vi "Configure Server.vi"(8 "error in (no error)":errorcluster, 9 "server configuration":cluster{"enabled":bool}, 10 "server index":u16, 11 "PLBB in":refnum<class "PL BlackBox Modbus Client.lvclass">) -> (0 "error out":errorcluster, 3 "PLBB out":refnum<class "PL BlackBox Modbus Client.lvclass">)   [LabVIEW 2015, in "PL BlackBox Modbus Client.lvclass"]
doc: "Configures the server."
uses:
  PL BlackBox Modbus Client.lvclass
  <vilib>/plasmapper/PL Modbus Client/PL Modbus Client.lvclass
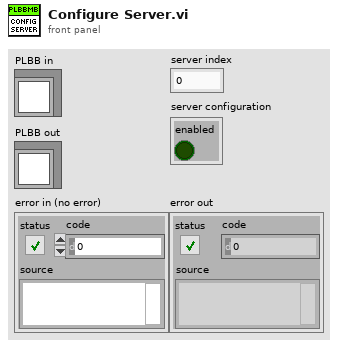
[diagram p1: front panel]
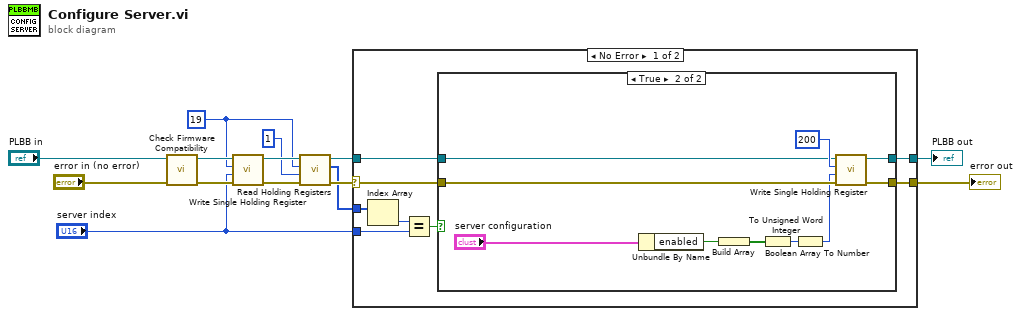
[diagram p0: block diagram]
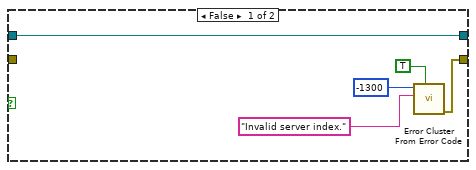
[diagram p2: hidden frame]
diagram:
  w6 = u16 19 ("address")
  n1 = call-dynamic "Check Firmware Compatibility.vi"("error in (no error)"="error in (no error)", "PLBB in"="PLBB in") -> ("error out"=w9:errorcluster, "PLBB out"=w10:refnum<class "PL BlackBox Modbus Client.lvclass">)  [unwired: 8 in]
  n2 = call <vilib>:"Write Single Holding Register.vi"("error in (no error)"=w9, "value"="server index", "address"=w6, "MODBUS in"=w10) -> ("error out"=w5:errorcluster, "MODBUS out"=w8:refnum<class "PL BlackBox Modbus Client.lvclass">)  [unwired: 6 in]
  n3 = call <vilib>:"Read Holding Registers.vi"("error in (no error)"=w5, "number of holding registers"=u16 1 ("address"), "address"=w6, "MODBUS in"=w8) -> ("error out"=w4:errorcluster, "values"=w2:u16[], "MODBUS out"=w3:refnum<class "PL BlackBox Modbus Client.lvclass">)  [unwired: 5 in]
  n4 = case shown="No Error" w4 {
    selector: w4 -> [w16 w38]
    tunnel: [w22 w38] -> w14
    tunnel: [w21 w39] -> w13
    tunnel: w3 -> [w17 w39]
    tunnel: w2 -> [w20 _]
    tunnel: "server index" -> [w15 _]
    frame No Error {
      n5 = Index Array(array=w20) -> (element=w19:u16)  [unwired: 1 in]
      n6 = Equal?(x=w19, y=w15) -> (x = y?=w18:bool)
      n7 = case shown="True" w18 {
        tunnel: [w23 w36] -> w22
        tunnel: [w27 w37] -> w21
        tunnel: w17 -> [w27 w30]
        tunnel: w16 -> [_ w29]
        frame False {
          n8 = call <vilib>:"Error Cluster From Error Code.vi"("show call chain? (False)"=TRUE, "error message (\"\")"="Invalid server index." ("error message (\"\")"), "error code (0)"=-1300) -> ("error out"=w23:errorcluster)  [unwired: 6 in]
        }
        frame True {
          n9 = Unbundle By Name("server configuration") -> ("enabled"=w33:bool)
          n10 = Build Array(w33) -> (w32:bool[])
          n11 = Boolean Array To Number(Boolean array=w32) -> (number=w31:u32)
          n12 = To Unsigned Word Integer(number=w31) -> (unsigned 16bit integer=w28:u16)
          n13 = call <vilib>:"Write Single Holding Register.vi"("error in (no error)"=w29, "value"=w28, "address"=u16 200, "MODBUS in"=w30) -> ("error out"=w36:errorcluster, "MODBUS out"=w37:refnum<class "PL BlackBox Modbus Client.lvclass">)  [unwired: 6 in]
        }
      }
    }
    frame Error {
    }
  }
  "error out" <- w14
  "PLBB out" <- w13
